vi "DSB Modulation Demo (Baseband-Sine) - Squared.vi"() -> ()   [LabVIEW 2013]
uses:
  <vilib>/express/express analysis/Spectral/Block/exnSpectralBlock spectral measurements RMS poly.vi
  <vilib>/express/express analysis/Spectral/Block/exnSpectralBlock spectral measurements RMS DDT.vi
  <vilib>/express/express analysis/Spectral/Block/exnSpectralBlock spectral measurements power poly.vi
  <vilib>/express/express analysis/Spectral/Block/exnSpectralBlock spectral measurements power DDT.vi
  <vilib>/express/express analysis/Spectral/XNode/ExpressSpectralMeasurementsBlockNode.xnode
panel:
  out "Estimated Freq":dbl
  in  "Modulation Freq.":dbl=2000.0 caption="Frequency"
  in  "?":enum32{"DSB FFT", "DSB Squared"}(tab)
  out "DSB FFT":dynamicdata(graph)
  out "DSB Squared":dynamicdata(graph)
  in  "WAV Sample Rate":dbl=44100.0 caption="dt"
  in  "LPF Cut-Off":dbl=10000.0 caption="Lower Cut-Off"
  in  "SNR (dB)":dbl(slide)=30.0 caption="Standard deviation" scale=-20.0..30.0
  out "Comparision":dynamicdata(graph)
  out "Baseband":dynamicdata(graph)
  out "DSB Wave":dynamicdata(graph)
  in  "Carrier Amp.":dbl=1.0 caption="Amplitude"
  in  "stop":bool
  in  "Frequency Offset":dbl(slide) scale=0.0..1000.0
  in  "Carrier Freq.":dbl=100000.0 caption="Frequency"
  # "DSB Modulation"
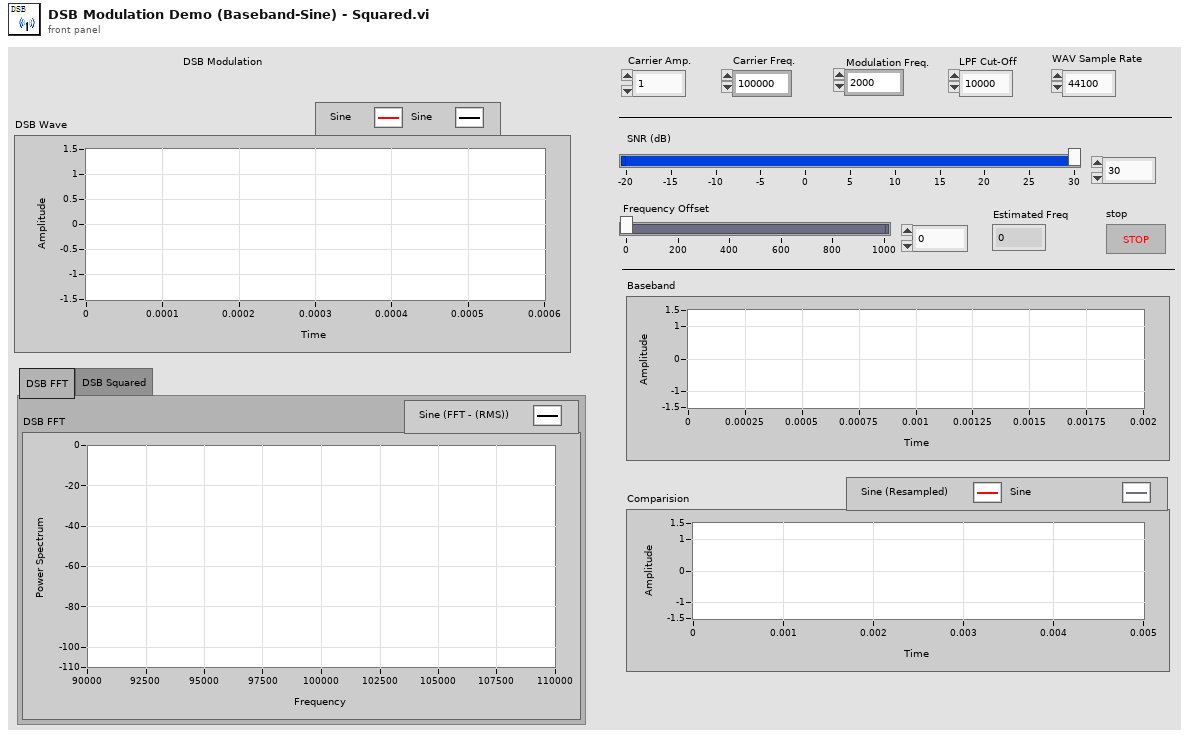
[diagram p1: front panel]
types:
  T1 = cluster{"averaging mode":u16, "weighting mode":u16, "number of averages":u32}
  T2 = cluster{"dB On (F)":bool, "unwrap phase (F)":bool, "convert to degree (F)":bool}
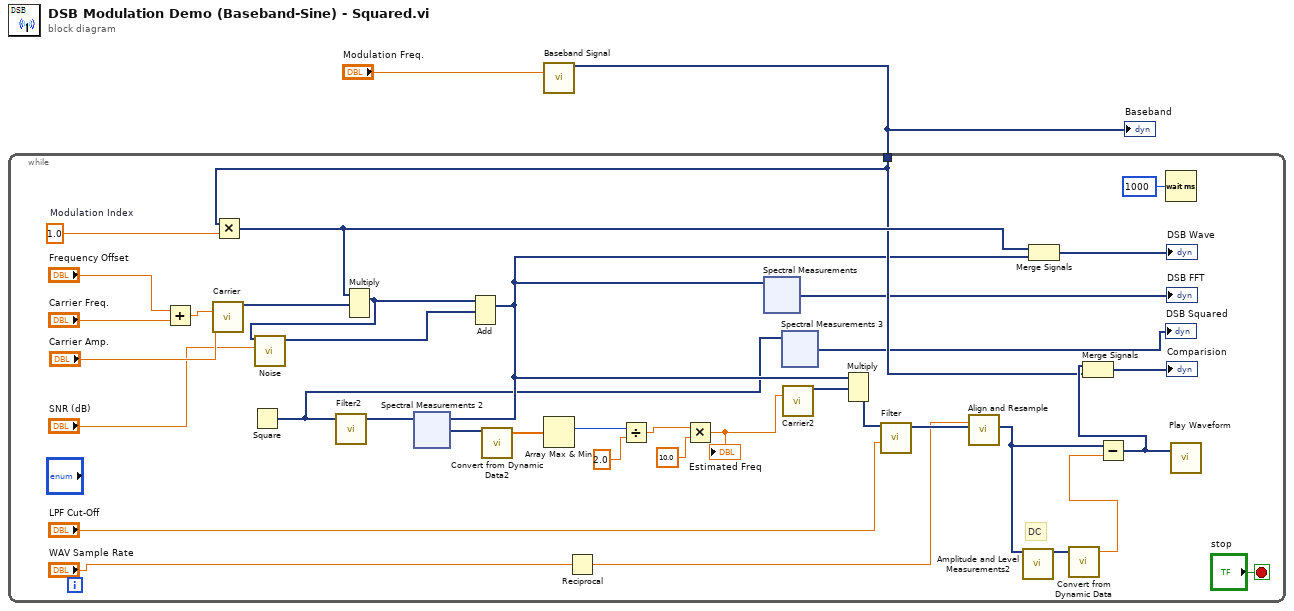
[diagram p0: block diagram]
diagram:
  n1 = call "Baseband Signal"("Frequency"="Modulation Freq.") -> ("Sine"=w1:dynamicdata)  [unwired: 13 in, 1 out]
  "Baseband" <- w1
  n2 = while {
    tunnel: w1 -> [w20]
    stop <- "stop" stop-if-true
    w33 = 1.0  # Modulation Index
    # "DC"
    n3 = Add(x="Frequency Offset", y="Carrier Freq.") -> (x+y=w32:dbl)
    n4 = call "Carrier"("Frequency"=w32, "Amplitude"="Carrier Amp.") -> ("Sine"=w30:dynamicdata)  [unwired: 12 in, 1 out]
    n5 = Multiply(x=w20, y=w33) -> (x*y=w29:dynamicdata)
    n6 = Multiply(1:w30, 2:w29) -> (0:w15:dynamicdata)  [unwired: 1 in, 1 out]
    n7 = call "Noise.vi"("AWGN (dB)"="SNR (dB)", "Dynamic Data"=w15) -> ("DC with Gaussian Noise"=w28:dynamicdata)  [unwired: 9 in]
    n8 = Add(1:w28, 2:w15) -> (0:w14:dynamicdata)  [unwired: 1 in, 1 out]
    n9 = Square(x=w14) -> (x^2=w13:dynamicdata)
    n10 = call "Filter2"("Signal"=w13) -> ("Filtered Signal"=w10:dynamicdata)  [unwired: 9 in, 1 out]
    n11 = xnode "Spectral Measurements 2"("Signals"=w10) -> ("Power Spectrum"=w9:dynamicdata)  [unwired: 1 in, 1 out]
    n12 = call "Convert from Dynamic Data2"("Dynamic Data Type"=w9) -> ("Array"=w8:dbl[])  [unwired: 3 in]
    n13 = Array Max & Min(array=w8) -> (max index (indices)=w7:i32)  [unwired: 3 out]
    n14 = Reciprocal(x="WAV Sample Rate") -> (1/x=w16:dbl)
    n15 = Divide(x=w7, y=2.0) -> (x/y=w5:dbl)
    n16 = Multiply(x=w5, y=10.0) -> (x*y=w3:dbl)
    "Estimated Freq" <- w3
    n17 = xnode "Spectral Measurements"("Signals"=w14) -> ("FFT - (RMS)"=→"DSB FFT":dynamicdata)  [unwired: 2 in, 3 out]
    n18 = xnode "Spectral Measurements 3"("Signals"=w13) -> ("FFT - (RMS)"=→"DSB Squared":dynamicdata)  [unwired: 2 in, 3 out]
    n19 = call "Carrier2"("Frequency"=w3) -> ("Sine"=w25:dynamicdata)  [unwired: 13 in, 1 out]
    n20 = Multiply(1:w25, 2:w14) -> (0:w24:dynamicdata)  [unwired: 1 in, 1 out]
    n21 = call "Filter"("Lower Cut-Off"="LPF Cut-Off", "Signal"=w24) -> ("Filtered Signal"=w23:dynamicdata)  [unwired: 8 in, 1 out]
    n22 = call "Align and Resample"("dt"=w16, "Signals"=w23) -> ("Resampled Signals"=w36:dynamicdata)  [unwired: 7 in, 2 out]
    n23 = call "Amplitude and Level Measurements2"("Signals"=w36) -> ("Mean (DC)"=w38:dynamicdata)  [unwired: 13 in, 1 out]
    n24 = Merge Signals(w29, w14) -> (→"DSB Wave":dynamicdata)
    n25 = call "Convert from Dynamic Data"("Dynamic Data Type"=w38) -> ("Scalar"=w35:dbl)  [unwired: 3 in]
    n26 = Subtract(x=w36, y=w35) -> (x-y=w21:dynamicdata)
    n27 = Merge Signals(w21, w20) -> (→"Comparision":dynamicdata)
    n28 = Wait (ms)(milliseconds to wait=u32 1000) -> ()  [unwired: 1 out]
    n29 = call "Play Waveform"("Data"=w21) -> ()  [unwired: 18 in, 1 out]
  }
